vi "Refresh Create Listbox Row.vi"(7 "Refresh Symbol (Blank)":T2, 8 "Change? (T)":bool=TRUE, 9 "New Item":string, 10 "Old Item":string, 11 "Refresh Listbox":T1) -> (3 "Refresh Listbox out":T1)   [LabVIEW 2020, in "Communication Bus Template System Explorer.lvlib" / "Implementation.lvlib"]
uses:
  Implementation.lvlib
  Types/Refresh Symbols.ctl
  Types/Refresh Listbox.ctl
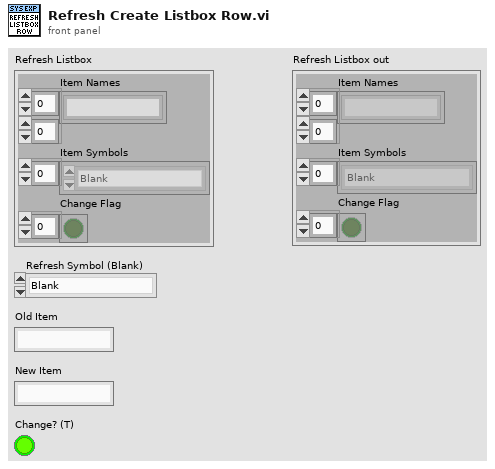
[diagram p1: front panel]
types:
  T1 = typedef "Communication Bus Template System Explorer.lvlib/Implementation.lvlib/Refresh Listbox.ctl" = cluster{"Item Names":string[][], "Item Symbols":T2[], "Change Flag":bool[]}
  T2 = typedef "Communication Bus Template System Explorer.lvlib/Implementation.lvlib/Refresh Symbols.ctl" = enum16{"Blank", "Port", "Incoming", "Outgoing", "Frame", "Signal", "Cluster", "Baud Rate"}
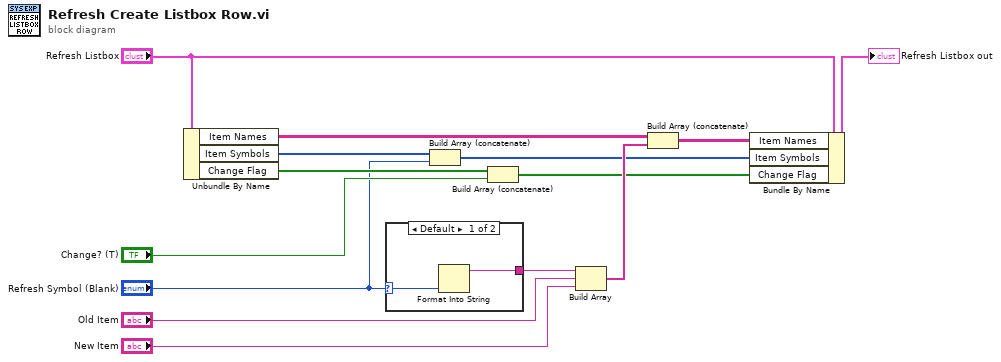
[diagram p0: block diagram]
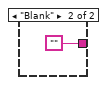
[diagram p2: hidden frame]
diagram:
  n1 = Unbundle By Name("Refresh Listbox") -> ("Item Names"=w8:string[][], "Item Symbols"=w7:T2[], "Change Flag"=w4:bool[])
  n2 = case shown="Default" "Refresh Symbol (Blank)" {
    selector: "Refresh Symbol (Blank)" -> [w15 _]
    tunnel: [w16 ""] -> w14
    frame Default {
      n3 = Format Into String(w15) -> (resulting string=w16:string)  [unwired: 3 in, 1 out]
    }
    frame "Blank" {
    }
  }
  n4 = Build Array (concatenate)(w7, "Refresh Symbol (Blank)") -> (w5:T2[])
  n5 = Build Array (concatenate)(w4, "Change? (T)") -> (w2:bool[])
  n6 = Build Array(w14, "Old Item", "New Item") -> (w11:string[])
  n7 = Build Array (concatenate)(w8, w11) -> (w6:string[][])
  n8 = Bundle By Name(cluster="Refresh Listbox", "Item Names"=w6, "Item Symbols"=w5, "Change Flag"=w2) -> (→"Refresh Listbox out":T1)
